vi "getOptionsString.vi"(8 "error in (no error)":errorcluster, 11 "tBSONRegEx in":refnum<class "tBSONRegEx.lvclass">) -> (0 "error out":errorcluster, 2 "OptionsString":string, 3 "tBSONRegEx out":refnum<class "tBSONRegEx.lvclass">)   [LabVIEW 2013, in "BSON.lvlib" / "tBSONRegEx.lvclass"]
uses:
  tBSONRegEx.lvclass
  tBSONRegEx.lvclass/tBSONRegEx.ctl
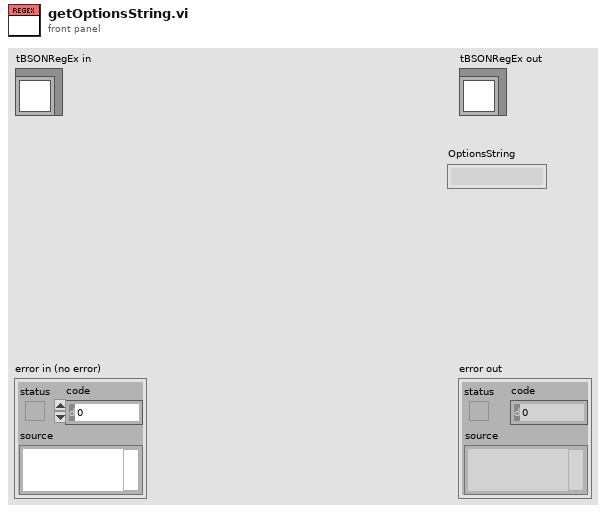
[diagram p1: front panel]
types:
  T1 = cluster{"Case Insensitive":bool, "Multiple Matching":bool, "Verbose Mode":bool, "Make \\w, \\W Local Dependent":bool, "Dotall mode":bool, "Make \\w, \\W Match Unicode":bool}
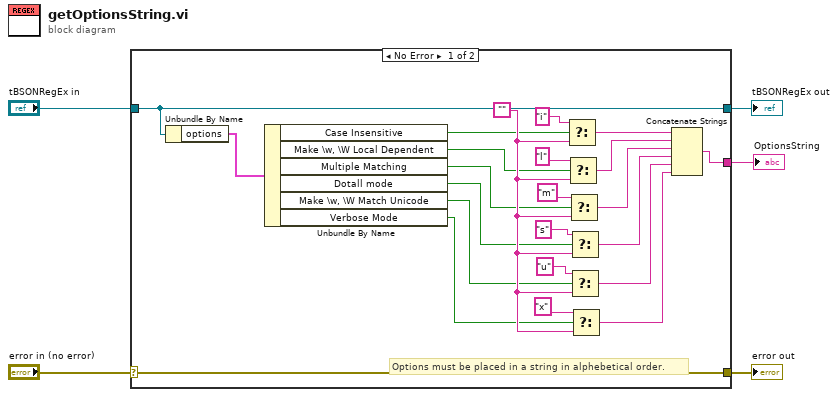
[diagram p0: block diagram]
diagram:
  n1 = case shown="No Error" "error in (no error)" {
    selector: "error in (no error)" -> [w28 w30]
    tunnel: [w28 w30] -> w4
    tunnel: [w27 w29] -> w2
    tunnel: "tBSONRegEx in" -> [w27 w29]
    tunnel: [w6 _] -> w1
    frame No Error {
      w20 = ""
      # "Options must be placed in a string in alphebetical order."
      n2 = Unbundle By Name(w27) -> ("options"=w7:T1)
      n3 = Unbundle By Name(w7) -> ("Case Insensitive"=w13:bool, "Make \\w, \\W Local Dependent"=w12:bool, "Multiple Matching"=w11:bool, "Dotall mode"=w10:bool, "Make \\w, \\W Match Unicode"=w9:bool, "Verbose Mode"=w8:bool)
      n4 = Select(t="i", s=w13, f=w20) -> (s? t:f=w26:string)
      n5 = Select(t="l", s=w12, f=w20) -> (s? t:f=w25:string)
      n6 = Select(t="m", s=w11, f=w20) -> (s? t:f=w24:string)
      n7 = Select(t="s", s=w10, f=w20) -> (s? t:f=w23:string)
      n8 = Select(t="u", s=w9, f=w20) -> (s? t:f=w21:string)
      n9 = Select(t="x", s=w8, f=w20) -> (s? t:f=w14:string)
      n10 = Concatenate Strings(w26, w25, w24, w23, w21, w14) -> (w6:string)
    }
    frame Error {
    }
  }
  "error out" <- w4
  "tBSONRegEx out" <- w2
  "OptionsString" <- w1
